vi "Add Link.vi"(0 "ParentLinkNode in":refnum<class "PanelLinkNode.lvclass"> caption="DNL_LabVIEW Object in", 1 "ChildNode* in":refnum<data-value>, 2 "L\\R Child":enum16{"LChild", "RChild"}(ring), 3 "error in (no error)":errorcluster caption="错误输入（无错误）") -> (7 "ParentLinkNode out":refnum<class "PanelLinkNode.lvclass"> caption="DNL_LabVIEW Object out", 10 "error out":errorcluster caption="错误输出")   [LabVIEW 2013, in "PanelLinkNode.lvclass"]
uses:
  PanelLinkNode.lvclass
  PanelObject/PanelObject.lvclass
  PanelLinkNode.lvclass/PanelLinkNode.ctl
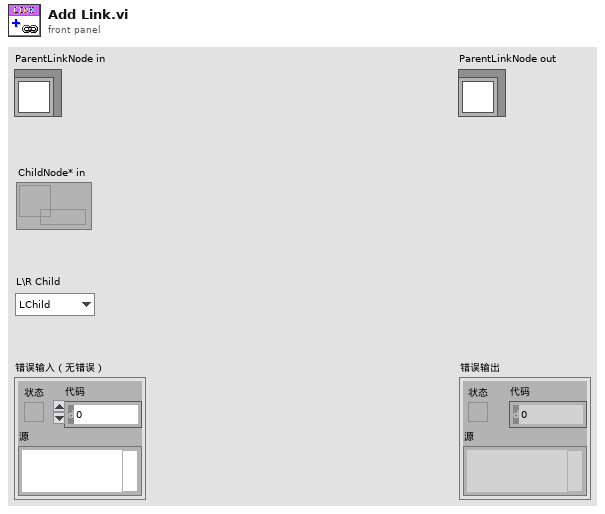
[diagram p1: front panel]
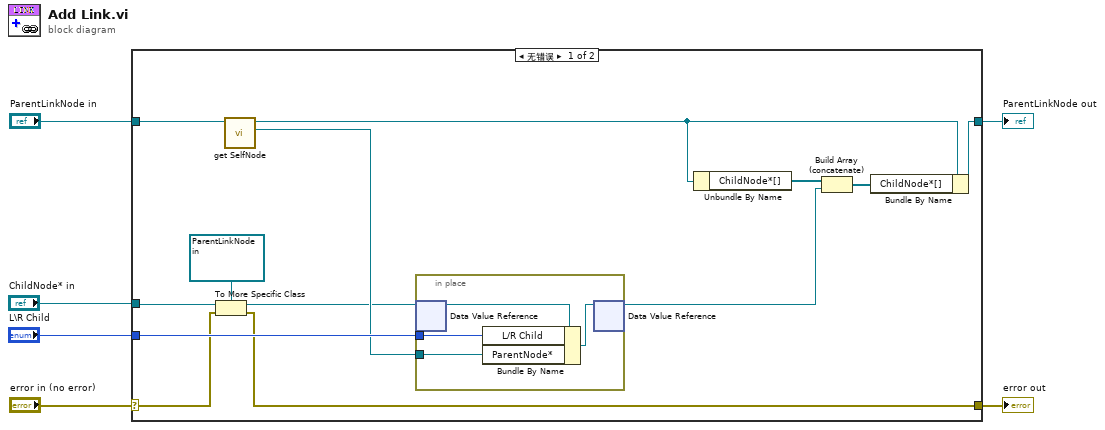
[diagram p0: block diagram]
diagram:
  n1 = case shown="无错误" "error in (no error)" {
    selector: "error in (no error)" -> [w12 w25]
    tunnel: [w11 w25] -> w5
    tunnel: [w9 w24] -> w4
    tunnel: "ParentLinkNode in" -> [w8 w24]
    tunnel: "L\\R Child" -> [w19 _]
    tunnel: "ChildNode* in" -> [w15 _]
    frame No Error {
      n2 = To More Specific Class(target class=refnum<data-value> refnum ("ChildNode* in"), reference=w15, error in=w12) -> (specific class reference=w13:refnum<data-value>, error out=w11:errorcluster)
      n3 = call "get SelfNode.vi"("PanelLinkNode输入"=w8) -> ("SelfNode*"=w18:refnum<data-value>, "PanelLinkNode输出"=w10:refnum<class "PanelLinkNode.lvclass">)  [unwired: 8 in, 1 out]
      n4 = in-place {
        in-place-border: w19 -> [w22]
        in-place-border: w18 -> [w20]
        n5 = in-place-dvr #1(w13) -> (w23:refnum<class "PanelLinkNode.lvclass">)  [unwired: 1 out]
        n6 = Bundle By Name(cluster=w23, "L/R Child"=w22, "ParentNode*"=w20) -> (w21:refnum<class "PanelLinkNode.lvclass">)
        n7 = in-place-dvr #1(w21) -> (w7:refnum<data-value>)  [unwired: 1 out]
      }
      n8 = Unbundle By Name(w10) -> ("ChildNode*[]"=w17:refnum<data-value>[])
      n9 = Build Array (concatenate)(w17, w7) -> (w16:refnum<data-value>[])
      n10 = Bundle By Name(cluster=w10, "ChildNode*[]"=w16) -> (w9:refnum<class "PanelLinkNode.lvclass">)
    }
    frame Error {
    }
  }
  "error out" <- w5
  "ParentLinkNode out" <- w4
